vi "HW_GEN - Generate Data Queue Info.vi"(8 "error in (no error)":errorcluster, 10 "DevInfo[]":T4[](array[typedef]), 11 "daqModuPara[]":T3(array[cluster])) -> (0 "error out":errorcluster, 2 "data queue[]":T1[](array[typedef]))   [LabVIEW 2016]
uses:
  Ctrls/HardWare _ Data Queue Info.ctl
  Ctrls/HardWare Basic Info _ Channel.ctl
  Ctrls/HardWare Basic Info _ Module.ctl
  Ctrls/HardWare Basic Info _ Chassis.ctl
  Ctrls/HardWare Basic Info _ Device.ctl
  Ctrls/HardWare _ Channel Parameters.ctl
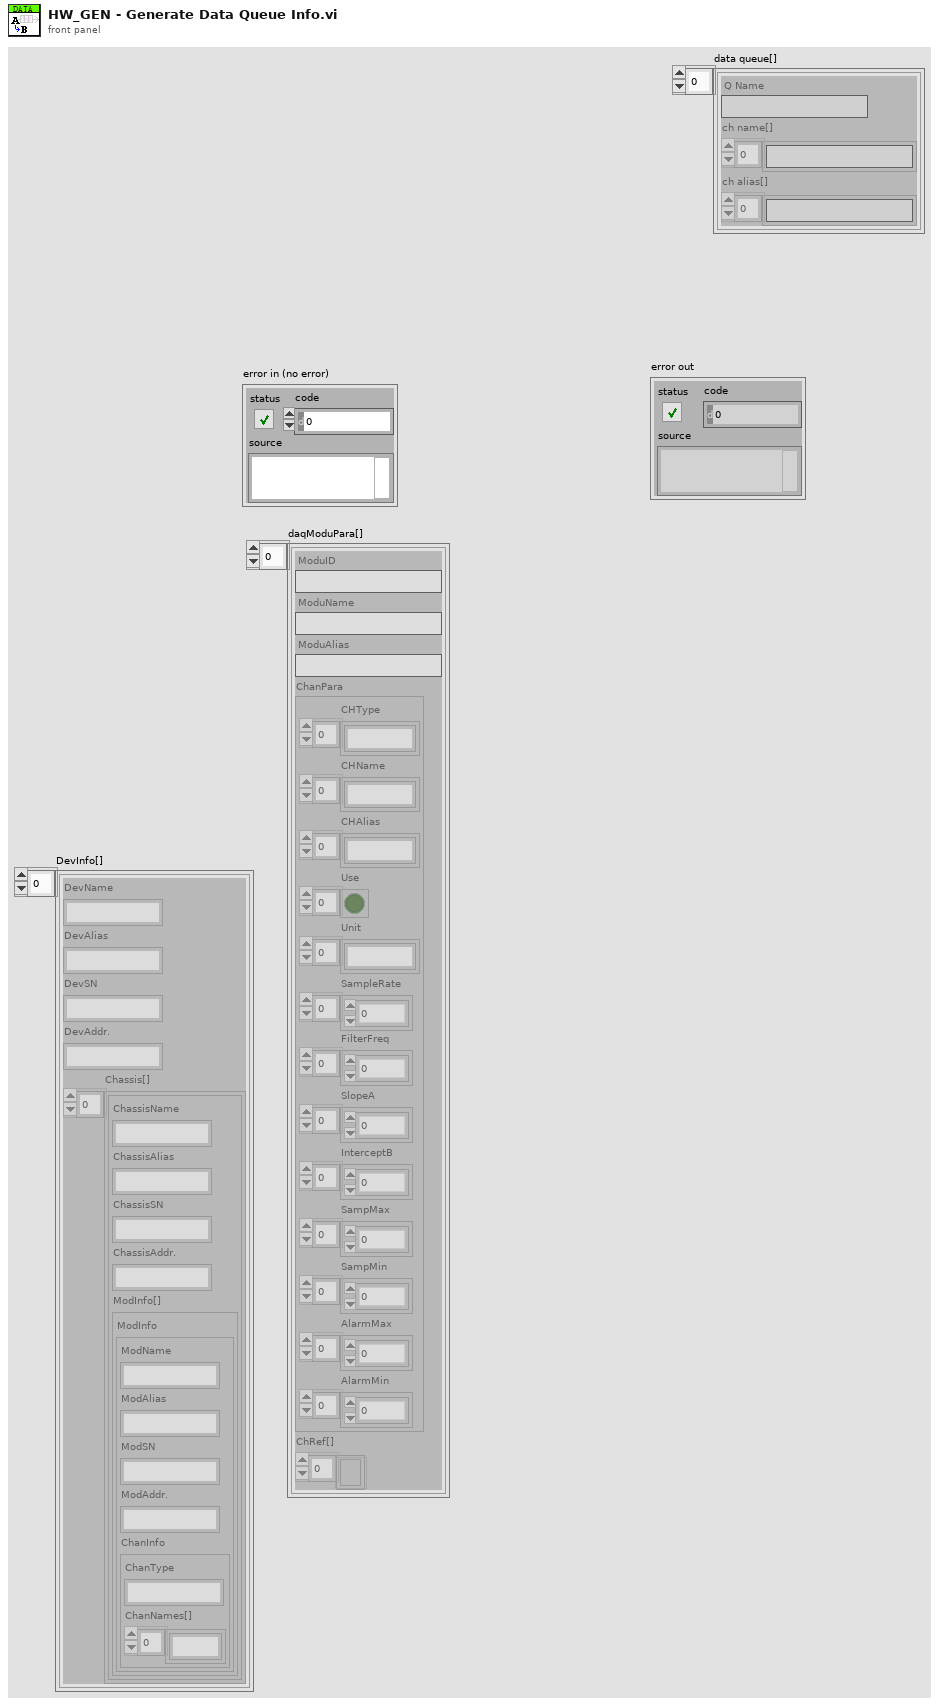
[diagram p1: front panel]
types:
  T1 = typedef "HardWare _ Data Queue Info.ctl" = cluster{"Q Name":string, "ch name[]":string[], "ch alias[]":string[]}
  T2 = typedef "HardWare _ Channel Parameters.ctl" = cluster{"CHType":string[], "CHName":string[], "CHAlias":string[], "Use":bool[], "Unit":string[], "SampleRate":dbl[], "FilterFreq":dbl[], "SlopeA":dbl[], "InterceptB":dbl[], "SampMax":dbl[], "SampMin":dbl[], "AlarmMax":dbl[], "AlarmMin":dbl[]}
  T3 = cluster{"ModuID":string, "ModuName":string, "ModuAlias":string, "ChanPara":T2, "ChRef[]":refnum<k24>[]}[]
  T4 = typedef "HardWare Basic Info _ Device.ctl" = cluster{"DevName":string, "DevAlias":string, "DevSN":string, "DevAddr.":string, "Chassis[]":T5[]}
  T5 = typedef "HardWare Basic Info _ Chassis.ctl" = cluster{"ChassisName":string, "ChassisAlias":string, "ChassisSN":string, "ChassisAddr.":string, "ModInfo[]":T6[]}
  T6 = typedef "HardWare Basic Info _ Module.ctl" = cluster{"ModName":string, "ModAlias":string, "ModSN":string, "ModAddr.":string, "ChanInfo":T7}
  T7 = typedef "HardWare Basic Info _ Channel.ctl" = cluster{"ChanType":string, "ChanNames[]":string[]}
  T8 = cluster{"ModuID":string, "ModuName":string, "ModuAlias":string, "ChanPara":T2, "ChRef[]":refnum<k24>[]}
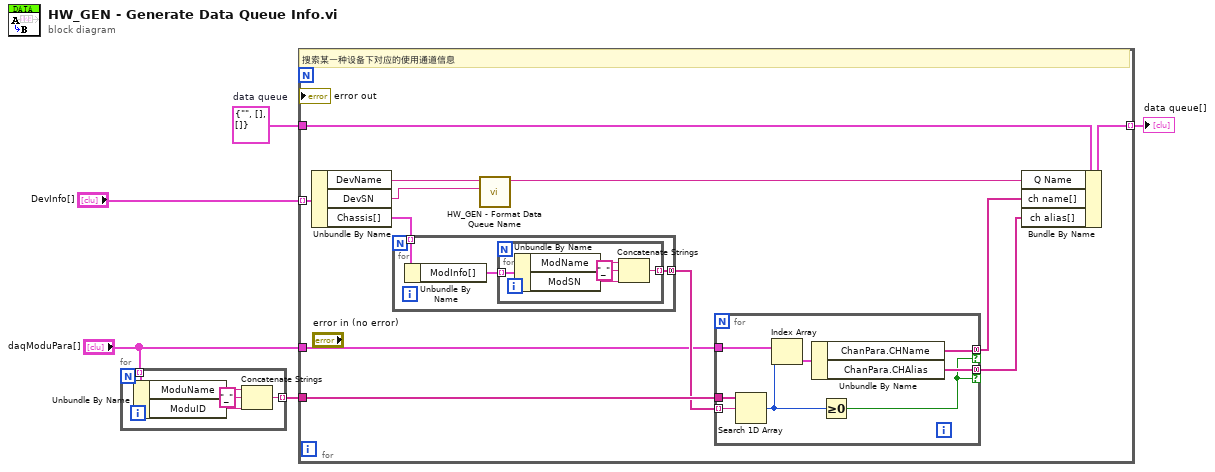
[diagram p0: block diagram]
diagram:
  w2 = T1 {"Q Name"="", "ch name[]"=[], "ch alias[]"=[]}  # data queue
  n1 = for {
    tunnel: "daqModuPara[]" -> [w10] mode=indexing
    tunnel: [w6] -> w4 mode=indexing
    n2 = Unbundle By Name(w10) -> ("ModuName"=w9:string, "ModuID"=w8:string)
    n3 = Concatenate Strings(w9, "_" ("string"), w8) -> (w6:string)
  }
  n4 = for {
    tunnel: "DevInfo[]" -> [w22] mode=indexing
    tunnel: w4 -> [w18]
    tunnel: "daqModuPara[]" -> [w16]
    tunnel: w2 -> [w15]
    tunnel: [w11] -> w1 mode=indexing
    # "搜索某一种设备下对应的使用通道信息"
    n5 = Unbundle By Name(w22) -> ("DevName"=w21:string, "DevSN"=w20:string, "Chassis[]"=w19:T5[])
    n6 = for {
      tunnel: w19 -> [w33] mode=indexing
      tunnel: [w31] -> w17 mode=concatenating
      n7 = Unbundle By Name(w33) -> ("ModInfo[]"=w32:T6[])
      n8 = for {
        tunnel: w32 -> [w38] mode=indexing
        tunnel: [w34] -> w31 mode=indexing
        n9 = Unbundle By Name(w38) -> ("ModName"=w37:string, "ModSN"=w36:string)
        n10 = Concatenate Strings(w37, "_" ("string"), w36) -> (w34:string)
      }
    }
    n11 = call "HW_GEN - Format Data Queue Name.vi"("DevSN"=w20, "DevName"=w21) -> ("Q Name"=w14:string)  [unwired: 9 in]
    n12 = for {
      tunnel: w18 -> [w30]
      tunnel: w17 -> [w29] mode=indexing
      tunnel: w16 -> [w28]
      tunnel: [w26] -> w13 mode=concatenating if=w23
      tunnel: [w25] -> w12 mode=concatenating if=w23
      n13 = Search 1D Array(1D array=w30, element=w29) -> (index of element=w24:i32)  [unwired: 1 in]
      n14 = Index Array(array=w28, index=w24) -> (element=w27:T8)
      n15 = Unbundle By Name(w27) -> ("ChanPara.CHName"=w26:string[], "ChanPara.CHAlias"=w25:string[])
      n16 = Greater Or Equal To 0?(x=w24) -> (x >= 0?=w23:bool)
    }
    n17 = Bundle By Name(cluster=w15, "Q Name"=w14, "ch name[]"=w13, "ch alias[]"=w12) -> (w11:T1)
  }
  "data queue[]" <- w1
